vi "ProcessArray.vi"(4 "Plot Data":bool, 6 "Aquire Data":bool, 8 "File Path In":path, 11 "array in":sgl[][](array[numeric])) -> (0 "file path out":path, 3 "Array out":T1(array[cluster]))   [LabVIEW 2020, in "SMU.lvclass"]
uses:
  SMU.lvclass
  <vilib>/Utility/file.llb/Write Delimited Spreadsheet (DBL).vi
  <vilib>/Analysis/NI_AALPro.lvlib
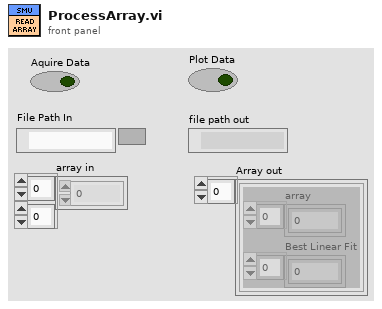
[diagram p1: front panel]
types:
  T1 = cluster{"array":sgl[], "Best Linear Fit":dbl[]}[]
  T2 = cluster{"array in":sgl[], "Best Linear Fit":dbl[]}
  T3 = cluster{"array in":sgl[], "Best Linear Fit":dbl[]}[]
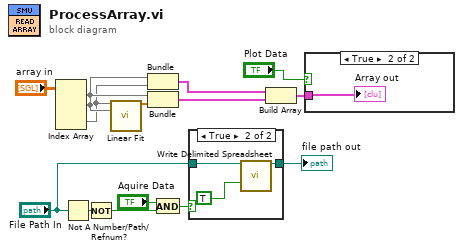
[diagram p0: block diagram]
diagram:
  n1 = Index Array(array="array in") -> (element #1=w7:sgl[], element #2=w6:sgl[])  [unwired: 4 in]
  n2 = Not A Number/Path/Refnum?(number/path/refnum="File Path In") -> (NaN/Path/Refnum?=w11:bool)
  n3 = Not(x=w11) -> (.not. x?=w12:bool)
  n4 = call <vilib>:"Linear Fit.vi"("Y"=w6, "X"=w7) -> ("Best Linear Fit"=w8:dbl[])  [unwired: 9 in, 4 out]
  n5 = Bundle("array in"=w7, "array in"=w6) -> (w4:cluster{"array in":sgl[], "array in":sgl[]})  [unwired: 1 in]
  n6 = Bundle("array in"=w7, "Best Linear Fit"=w8) -> (w5:T2)  [unwired: 1 in]
  n7 = And(x="Aquire Data", y=w12) -> (x .and. y?=w14:bool)
  n8 = case shown="True" w14 {
    tunnel: [w15 w17] -> w1
    tunnel: "File Path In" -> [w15 w18]
    frame False {
    }
    frame True {
      n9 = call-poly <vilib>:"Write Delimited Spreadsheet.vi"("file path (dialog if empty)"=w18, "append to file? (new file:F)"=TRUE) -> ("new file path (Not A Path if cancelled)"=w17:path)  [unwired: 12 in, 1 out]
    }
  }
  "file path out" <- w1
  n10 = Build Array(w4, w5) -> (w3:T3)
  n11 = case shown="True" "Plot Data" {
    tunnel: w3 -> [_ w19]
    frame False {
    }
    frame True {
      "Array out" <- w19
    }
  }
